vi "Board Player on Food.vi"(2 "Player":refnum<class "Player.lvclass">, 3 "Food":refnum<class "Food.lvclass">[](array[class])) -> (0 "Indices":i32[](array[numeric]), 1 "Found?":bool)   [LabVIEW 2019, in "Board.lvclass"]
uses:
  Board.lvclass
  Player/Player.lvclass
  Food/Food.lvclass
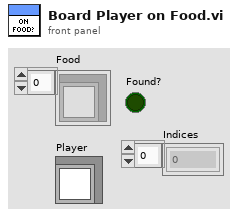
[diagram p1: front panel]
types:
  T1 = typedef "Coordinate STYP.ctl" = cluster{"X":i32, "Y":i32}
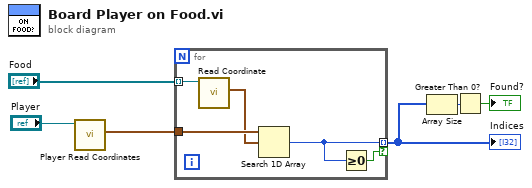
[diagram p0: block diagram]
diagram:
  n1 = call-dynamic "Player Read Coordinates.vi"("Player in"="Player") -> ("Coordinates"=w4:T1[])  [unwired: 8 in, 2 out]
  n2 = for {
    tunnel: "Food" -> [w10] mode=indexing
    tunnel: w4 -> [w11]
    tunnel: [w8] -> w1 mode=indexing if=w7
    n3 = call-dynamic "Read Coordinate.vi"("Food in"=w10) -> ("Coordinate"=w9:T1)  [unwired: 8 in, 2 out]
    n4 = Search 1D Array(1D array=w11, element=w9) -> (index of element=w8:i32)  [unwired: 1 in]
    n5 = Greater Or Equal To 0?(x=w8) -> (x >= 0?=w7:bool)
  }
  "Indices" <- w1
  n6 = Array Size(array=w1) -> (size(s)=w3:i32)
  n7 = Greater Than 0?(x=w3) -> (x > 0?=→"Found?":bool)
